vi "Server.vi"() -> ()   [LabVIEW 2021, in "Unary.lvlib"]
uses:
  Unary.lvlib
  TypeDef/Pin_Levels.ctl
  TypeDef/I2C_Bus_Timing.ctl
  <vilib>/gRPC/LabVIEW gRPC Library/Shared/grpcId.ctl
  Unary_server/RPC Service/I2C/I2C.lvclass
  <vilib>/gRPC/LabVIEW gRPC Servicer/Servicer/Servicer.lvclass/Servicer.ctl
  Unary_server/RPC Service/I2C/I2C.lvclass/I2C.ctl
  Unary_server/RPC Messages/Protocol_Response.ctl
  Unary_server/RPC Messages/Protocol_Request.ctl
  680a15a0-08d8-4a03-a66a-54d48a585acd.vi
  ed867548-5001-4521-8b76-5dbd51965f23.vi
  dd8acb0c-9aaa-46ce-9248-2d1e9a0b0157.vi
  <vilib>/JDP Science/JSONtext/JSON text to Variant.vi
  <vilib>/JDP Science/JSONtext/Variant to JSON Text.vi
  <vilib>/JDP Science/JSONtext/LVClass Serializer/JSONtext LVClass Serializer.lvclass
  <vilib>/gRPC/LabVIEW gRPC Servicer/Servicer/Servicer.lvclass
  Unary_server/Unary_server.lvlib
  <vilib>/gRPC/LabVIEW gRPC Library/grpc-lvsupport-release.lvlib
panel:
  in  "Server Address":string="localhost:50051"
  out "Configure I2C Bus timing":T1 {"Frequency(Hz)" min=10000.0 max=25000000.0 step=100.0 format="%#_6p"; "T_HD_DAT(ns)" step=1.0 format="%#_5g"; "T_SU_STA(ns)" min=0.0 step=1.0 format="%#_5g"; "T_HD_STA(ns)" min=0.0 step=1.0 format="%#_5g"; "T_SU_STO(ns)" min=0.0 step=1.0 format="%#_5g"; "T_BUF(ns)" min=0.0 step=1.0 format="%#_5g"; "T_HIGH(ns)" min=0.0 step=1.0 format="%#_5g"; "T_LOW(ns)" min=0.0 step=1.0 format="%#_5g"; "T_SU_DAT(ns)" step=1.0 format="%#_5g"}
  out "I2C Pin Levels":T2={"SCL VIH (V)"=0.0, "SCL VIL (V)"=0.0, "SCL Load Current (A)"=0.0015, "SDA VIH (V)"=0.0, "SDA VIL (V)"=0.0, "SDA Load Current (A)"=0.0015, "ModSeIL Termination Mode"="Internal", "ModSeIL VIL (V)"=0.0, "ModSeIL VIH (V)"=1.8} {"ModSeIL VIH (V)" min=-2.0 max=6.0 step=0.1 format="%#_2g"; "ModSeIL VIL (V)" min=-2.0 max=6.0 step=0.1 format="%#_2g"; "SDA Load Current (A)" min=0.0015 max=0.024 step=0.001 format="%#_2p"; "SDA VIH (V)" min=-2.0 max=6.0 step=0.1 format="%#_3g"; "SDA VIL (V)" min=-2.0 max=6.0 step=0.1 format="%#_3g"; "SCL Load Current (A)" min=0.0015 max=0.024 step=0.001 format="%#_2p"; "SCL VIH (V)" min=-2.0 max=6.0 step=0.1 format="%#_3g"; "SCL VIL (V)" min=-2.0 max=6.0 step=0.1 format="%#_3g"}
  out "Listening Port":i32=50051
  # "Unary Server"
  # "Pin Levels Configuration"
  # "SCL"
  # "SDA"
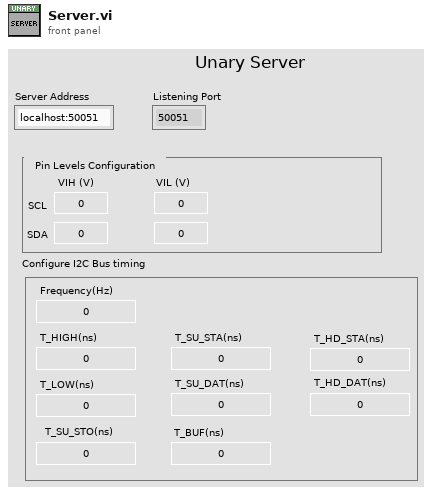
[diagram p1: front panel]
types:
  T1 = typedef "Unary.lvlib/I2C_Bus_Timing.ctl" = cluster{"Frequency(Hz)":dbl, "T_HIGH(ns)":dbl, "T_LOW(ns)":dbl, "T_SU_STO(ns)":dbl, "T_SU_STA(ns)":dbl, "T_SU_DAT(ns)":dbl, "T_BUF(ns)":dbl, "T_HD_STA(ns)":dbl, "T_HD_DAT(ns)":dbl}
  T2 = typedef "Unary.lvlib/Pin_Levels.ctl" = cluster{"SCL VIH (V)":dbl, "SCL VIL (V)":dbl, "SCL Load Current (A)":dbl, "SDA VIH (V)":dbl, "SDA VIL (V)":dbl, "SDA Load Current (A)":dbl, "ModSeIL Termination Mode":string, "ModSeIL VIL (V)":dbl, "ModSeIL VIH (V)":dbl}
  T3 = typedef "grpc-lvsupport-release.lvlib/grpcId.ctl" = u64
  T4 = typedef "Unary_server.lvlib/I2C.lvclass/Server gRPC UEs.ctl" = cluster{"I2C Configure gRPC UE":refnum<user-event>}
  T5 = typedef "Unary_server.lvlib/Protocol_Request.ctl" = cluster{"Request":string, "Data":string}
  T6 = typedef "Unary_server.lvlib/Protocol_Response.ctl" = cluster{"Operation":T5, "Status":bool}
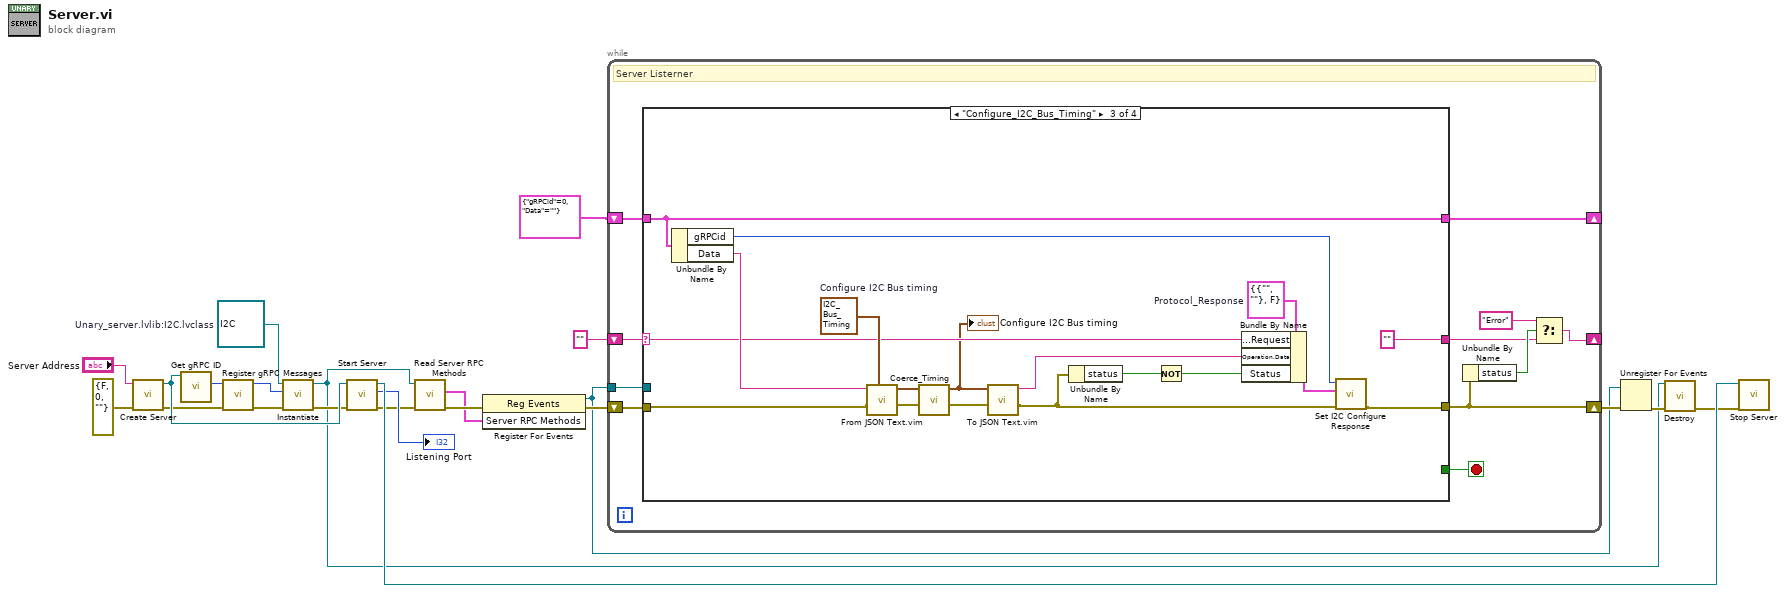
[diagram p0: block diagram]
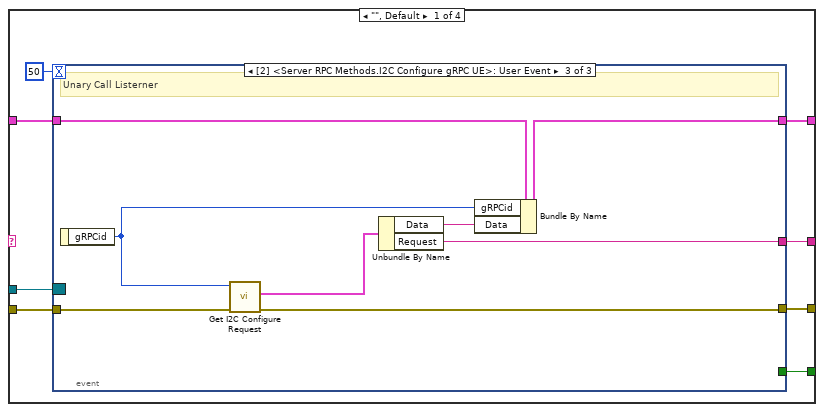
[diagram p2: hidden frame]
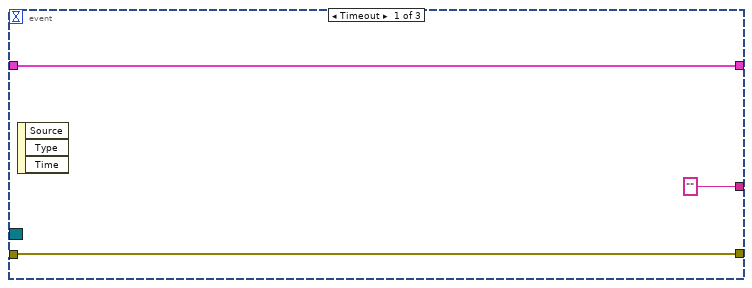
[diagram p3: hidden frame]
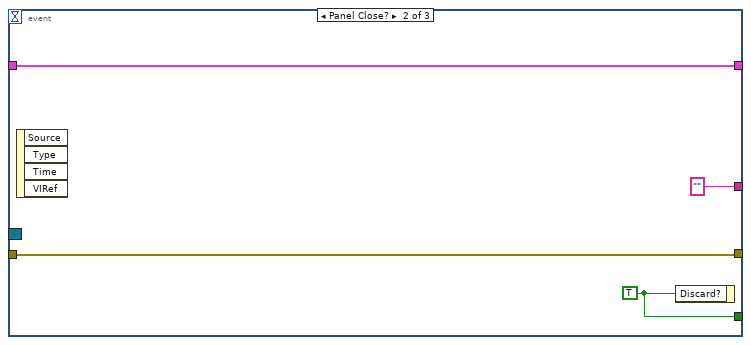
[diagram p4: hidden frame]
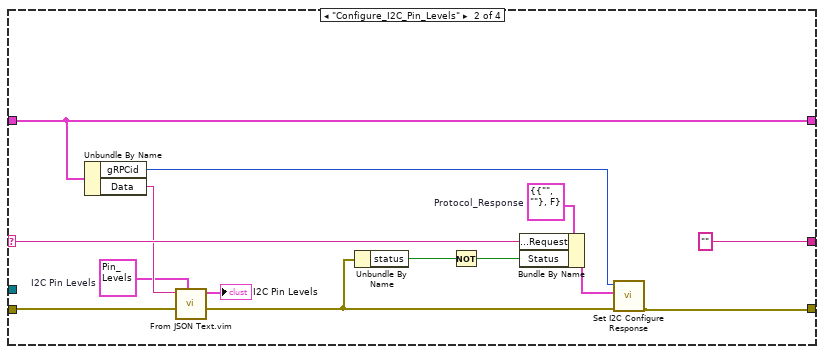
[diagram p5: hidden frame]
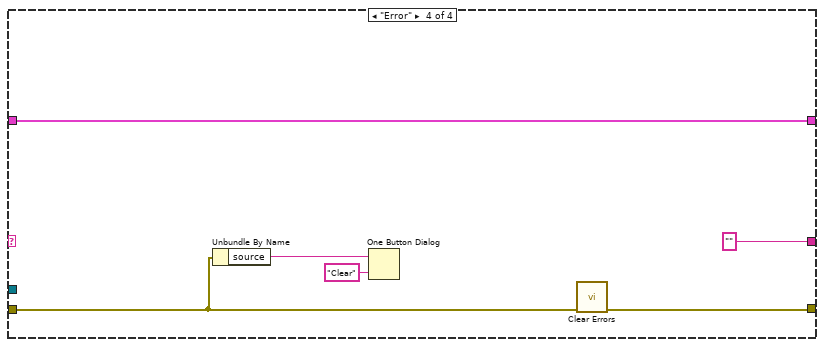
[diagram p6: hidden frame]
diagram:
  w1 = refnum<class "I2C.lvclass"> refnum  # Unary_server.lvlib:I2C.lvclass
  n1 = call <vilib>:"Create Server.vi"("error in"=errorcluster {"status"=FALSE, "code"=0, "source"=""} ("error in (no error)"), "Server Address"="Server Address") -> ("error out"=w7:errorcluster, "gRPC Server out"=w14:refnum<class "Servicer.lvclass">)  [unwired: 8 in]
  n2 = call <vilib>:"Get gRPC ID.vi"("OOP Server in"=w14) -> ("gRPC ID"=w8:T3)  [unwired: 9 in, 1 out]
  n3 = call "Register gRPC Messages.vi"("error in (no error)"=w7, "gRPC ID"=w8) -> ("error out"=w4:errorcluster, "gRPC ID Out"=w2:T3)  [unwired: 8 in]
  n4 = call-dynamic "Instantiate.vi"("error in"=w4, "gRPCid"=w2, "iService"=w1) -> ("error out"=w5:errorcluster, "iService"=w3:refnum<class "I2C.lvclass">)  [unwired: 7 in]
  n5 = call <vilib>:"Start Server.vi"("error in"=w5, "gRPC Server in"=w14) -> ("error out"=w9:errorcluster, "Listening Port"=→"Listening Port":i32, "gRPC Server out"=w16:refnum<class "Servicer.lvclass">)  [unwired: 7 in]
  n6 = call "Read Server RPC Methods.vi"("error in (no error)"=w9, "SignalGeneratorService in"=w3) -> ("error out"=w11:errorcluster, "Server RPC Methods"=w10:T4)  [unwired: 7 in, 1 out]
  n7 = register-events(error in=w11, w10) -> (reference out=w19:refnum<event-registration>, error out=w21:errorcluster)  [unwired: 1 in]
  n8 = while {
    shift-right: [w30] -> w20
    shift-left: w21 -> [w32]
    shift-right: [w28] -> _
    shift-left: "" -> [w33]
    tunnel: w19 -> [w25]
    shift-right: [w24] -> _
    shift-left: cluster{"gRPCid":T3, "Data":string} {"gRPCid"=0, "Data"=""} -> [w23]
    stop <- w31 stop-if-true
    # "Server Listerner"
    n9 = case shown="\"Configure_I2C_Bus_Timing\"" w33 {
      selector: w33 -> [_ w66 w73 _]
      tunnel: w32 -> [w41 w63 w77 w92]
      tunnel: [w40 w70 w87 w93] -> w30
      tunnel: [w39 "" ("Request") "" ("Request") ""] -> w27
      tunnel: [w38 _ _ _] -> w31
      tunnel: w25 -> [w36 _ _ _]
      tunnel: [w35 w69 w86 w88] -> w24
      tunnel: w23 -> [w34 w69 w86 w88]
      frame "", Default {
        n10 = event shown="[2] <Server RPC Methods.I2C Configure gRPC UE>: User Event" {
          selector: w36 -> [_ _ _]
          dyn-events: _ -> [_ _ _]
          timeout: 50 -> [_ _ _]
          tunnel: w41 -> [w44 w48 w56]
          tunnel: [w44 w48 w50] -> w40
          tunnel: ["" "" w54] -> w39
          tunnel: [_ w46 _] -> w38
          tunnel: [w42 w45 w52] -> w35
          tunnel: w34 -> [w42 w45 w53]
          event Timeout {
            n11 = event-data() -> ()  [unwired: 1 in, 3 out]
          }
          event Panel Close? {
            w46 = TRUE ("Discard?")
            n12 = event-data() -> ()  [unwired: 1 in, 4 out]
            n13 = event-data("Discard?"=w46) -> ()  [unwired: 1 in, 1 out]
          }
          event User Event {
            # "Unary Call Listerner"
            n14 = event-data() -> ("gRPCid"=w51:T3)  [unwired: 1 in]
            n15 = call "Get I2C Configure Request.vi"("error in (no error)"=w56, "gRPCid"=w51) -> ("error out"=w50:errorcluster, "Message Data"=w55:T5)  [unwired: 7 in, 1 out]
            n16 = Unbundle By Name(w55) -> ("Data"=w49:string, "Request"=w54:string)
            n17 = Bundle By Name(cluster=w53, "gRPCid"=w51, "Data"=w49) -> (w52:cluster{"gRPCid":T3, "Data":string})
          }
        }
      }
      frame "Configure_I2C_Pin_Levels" {
        w57 = T6 {"Operation"={"Request"="", "Data"=""}, "Status"=FALSE}  # Protocol_Response
        w61 = T2 {"SCL VIH (V)"=0.0, "SCL VIL (V)"=0.0, "SCL Load Current (A)"=0.0015, "SDA VIH (V)"=0.0, "SDA VIL (V)"=0.0, "SDA Load Current (A)"=0.0015, "ModSeIL Termination Mode"="Internal", "ModSeIL VIL (V)"=0.0, "ModSeIL VIH (V)"=1.8}  # I2C Pin Levels
        n18 = Unbundle By Name(w69) -> ("gRPCid"=w65:T3, "Data"=w62:string)
        n19 = call "From JSON Text.vim"("Data Type and Default Value"=w61, "error in (no error)"=w63, "JSON"=w62) -> ("error out"=w64:errorcluster, "Data out"=→"I2C Pin Levels":T2)  [unwired: 7 in]
        n20 = Unbundle By Name(w64) -> ("status"=w59:bool)
        n21 = Not(x=w59) -> (.not. x?=w58:bool)
        n22 = Bundle By Name(cluster=w57, "Operation.Request"=w66, "Status"=w58) -> (w67:T6)
        n23 = call "Set I2C Configure Response.vi"("error in (no error)"=w64, "Message Data"=w67, "gRPCid in"=w65) -> ("error out"=w70:errorcluster)  [unwired: 8 in]
      }
      frame "Configure_I2C_Bus_Timing" {
        w72 = T6 {"Operation"={"Request"="", "Data"=""}, "Status"=FALSE}  # Protocol_Response
        w79 = T1 {"Frequency(Hz)"=10000.0, "T_HIGH(ns)"=0.0, "T_LOW(ns)"=0.0, "T_SU_STO(ns)"=0.0, "T_SU_STA(ns)"=0.0, "T_SU_DAT(ns)"=0.0, "T_BUF(ns)"=0.0, "T_HD_STA(ns)"=0.0, "T_HD_DAT(ns)"=0.0}  # Configure I2C Bus timing
        n24 = Unbundle By Name(w86) -> ("gRPCid"=w83:T3, "Data"=w76:string)
        n25 = call "From JSON Text.vim"("Data Type and Default Value"=w79, "error in (no error)"=w77, "JSON"=w76) -> ("error out"=w78:errorcluster, "Data out"=w80:T1)  [unwired: 7 in]
        n26 = call "Coerce_Timing.vi"("Timing_In"=w80) -> ("Timing_Out"=w71:T1)  [unwired: 10 in]
        "Configure I2C Bus timing" <- w71
        n27 = call "To JSON Text.vim"("error in (no error)"=w78, "Anything"=w71) -> ("error out"=w82:errorcluster, "<JSON>"=w81:string)  [unwired: 8 in]
        n28 = Unbundle By Name(w82) -> ("status"=w75:bool)
        n29 = Not(x=w75) -> (.not. x?=w74:bool)
        n30 = Bundle By Name(cluster=w72, "Operation.Request"=w73, "Operation.Data"=w81, "Status"=w74) -> (w84:T6)
        n31 = call "Set I2C Configure Response.vi"("error in (no error)"=w82, "Message Data"=w84, "gRPCid in"=w83) -> ("error out"=w87:errorcluster)  [unwired: 8 in]
      }
      frame "Error" {
        n32 = Unbundle By Name(w92) -> ("source"=w90:string)
        n33 = One Button Dialog(message=w90, button name ("OK")="Clear") -> ()  [unwired: 1 out]
        n34 = call <vilib>:"Clear Errors.vi"("error in (no error)"=w92) -> ("error out"=w93:errorcluster)  [unwired: 5 in, 1 out]
      }
    }
    n35 = Unbundle By Name(w30) -> ("status"=w29:bool)
    n36 = Select(t="Error", s=w29, f=w27) -> (s? t:f=w28:string)
  }
  n37 = Unregister For Events(event registration refnum=w19, error in=w20) -> (error out=w12:errorcluster)
  n38 = call-dynamic "Destroy.vi"("error in (no error)"=w12, "SignalGeneratorService in"=w3) -> ("error out"=w13:errorcluster)  [unwired: 8 in, 1 out]
  n39 = call <vilib>:"Stop Server.vi"("error in"=w13, "gRPC Server in"=w16) -> ()  [unwired: 9 in, 1 out]
